vi "New Stuff.vi"(0 "Variant":variant, 1 "Variant 2":variant, 2 "Variant 4":variant, 3 "Variant 3":variant, 4 "Variant 16":variant, 5 "Variant 15":variant, 6 "Variant 8":variant, 7 "Variant 7":variant, 8 "Variant 5":variant, 9 "Variant 14":variant, 10 "Variant 12":variant, 11 "Variant 13":variant, 12 "Variant 11":variant, 13 "Variant 6":variant, 14 "Variant 10":variant, 15 "Variant 9":variant) -> (23 "x != y?":bool)   [LabVIEW 2018]
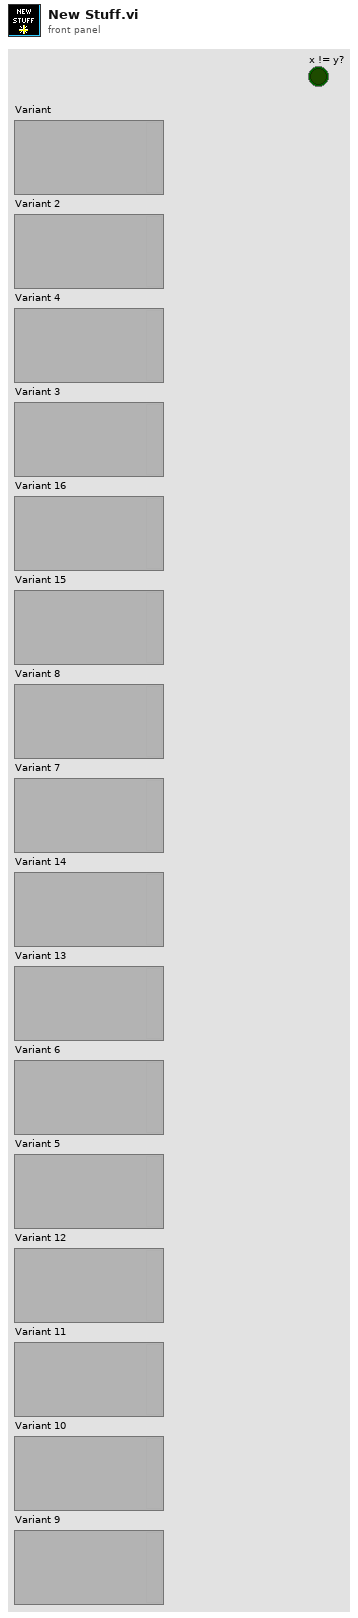
[diagram p1: front panel]
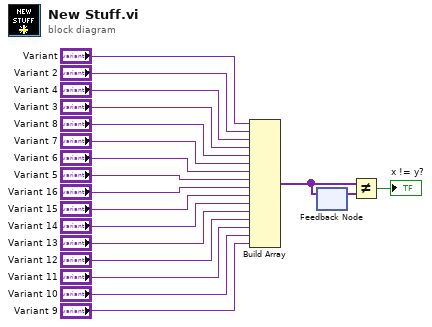
[diagram p0: block diagram]
diagram:
  n1 = Build Array("Variant", "Variant 2", "Variant 4", "Variant 3", "Variant 8", "Variant 7", "Variant 6", "Variant 5", "Variant 16", "Variant 15", "Variant 14", "Variant 13", "Variant 12", "Variant 11", "Variant 10", "Variant 9") -> (w1:variant[])
  n2 = feedback-in #1(w1) -> ()
  n3 = feedback #1() -> (w19:variant[])  [unwired: 1 in]
  n4 = Not Equal?(x=w1, y=w19) -> (x != y?=→"x != y?":bool)
